vi "Firmware Wizard Config.vi"(8 "Error In":errorcluster) -> (0 "Error Out":errorcluster)   [LabVIEW 2020, in "LMH-LINX.lvlib"]
doc: "Allow user to configure settings stored in firmware wizard ini."
uses:
  LMH-LINX.lvlib
  <vilib>/Utility/config.llb/Read Key (Path).vi
  <vilib>/Utility/config.llb/Write Key (Path).vi
  <vilib>/Utility/config.llb/NI_LVConfig.lvlib
  Toolbox/LMH-Toolbox.lvlib
panel:
  in  "Generate Firmware Libs":bool
  in  "Arduino Path":path
  in  "Cancel Button":bool
  in  "Save Button":bool
  in  "Firmware Base Path":path
  # "Default Location: <LabVIEW>\\vi.lib\\MakerHub\\LINX\\Firmware\\"
  # "Default Location: <Program Files (x86)>\\Arduino"
  # "If you have the Arduino IDE, fill in the Arduino Path and use the Generate button to Generate the  firmware in the Arduino\\libraries folder\nNOTE: This will erase existing firmware in this folder"
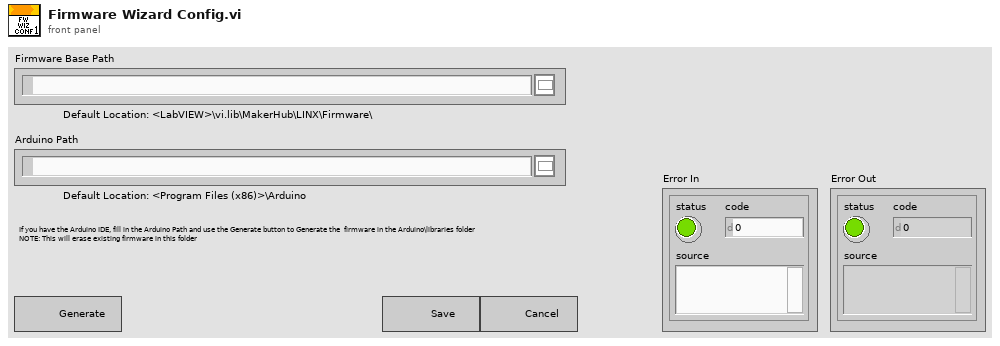
[diagram p1: front panel]
types:
  T1 = typedef "NI_LVConfig.lvlib/Config Data RefNum.ctl" = refnum<k1>
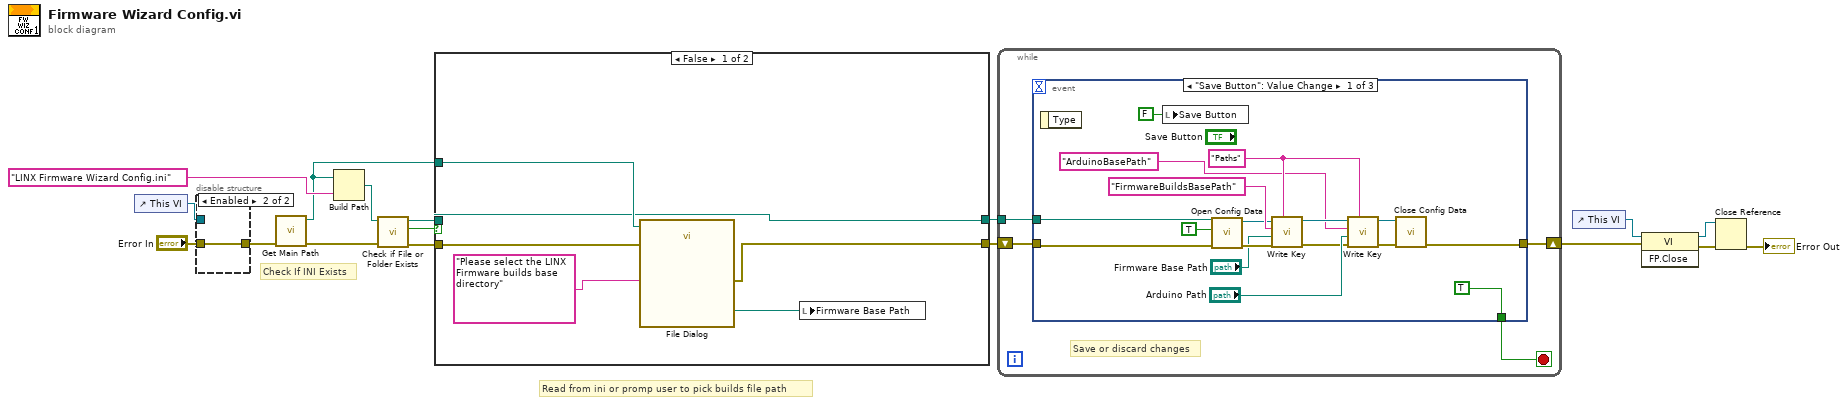
[diagram p0: block diagram]
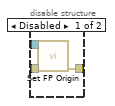
[diagram p2: hidden frame]
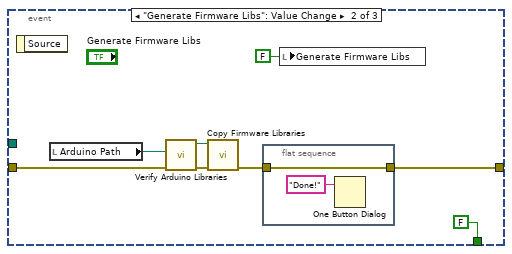
[diagram p3: hidden frame]
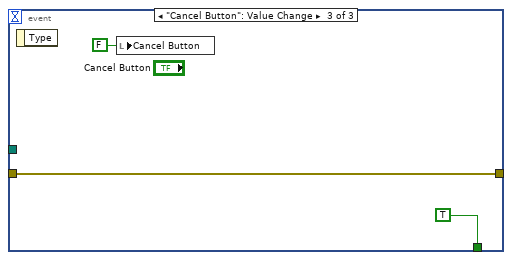
[diagram p4: hidden frame]
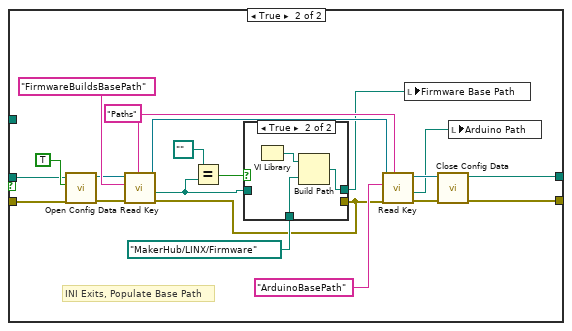
[diagram p5: hidden frame]
diagram:
  # "Read from ini or promp user to pick builds file path"
  # "Check If INI Exists"
  n1 = control-ref of="This VI"() -> (w8:refnum<vi>)
  n2 = disable-structure shown="Enabled" {
    disable-tunnel: w8 -> [w20 _]
    disable-tunnel: "Error In" -> [w19 w21]
    disable-tunnel: [w18 w21] -> w1
    frame Disabled {
      n3 = call <vilib>:"Set FP Origin.vi"("Error In"=w19, "VI Ref"=w20) -> ("Error Out"=w18:errorcluster)  [unwired: 9 in]
    }
    frame Enabled {
    }
  }
  n4 = call "Get Main Path.vi"("Error In"=w1) -> ("Error Out"=w16:errorcluster, "Main Dir"=w11:path)  [unwired: 8 in, 1 out]
  n5 = Build Path(base path=w11, name or relative path="LINX Firmware Wizard Config.ini") -> (appended path=w15:path)
  n6 = call <vilib>:"Check if File or Folder Exists.vi"("error in (no error)"=w16, "path"=w15) -> ("error out"=w12:errorcluster, "file or folder exists?"=w13:bool, "dup path"=w14:path)  [unwired: 7 in]
  n7 = case shown="False" w13 {
    tunnel: [w26 w43] -> w10
    tunnel: w14 -> [w24 w42]
    tunnel: w12 -> [w27 w41]
    tunnel: w11 -> [w25 _]
    tunnel: [w24 w40] -> w9
    frame False {
      n8 = call "File Dialog"("start path"=w25, "prompt"="Please select the LINX Firmware builds base directory", "error in"=w27) -> ("selected path"=w23:path, "error out"=w26:errorcluster)  [unwired: 9 in, 2 out]
      n9 = local write "Firmware Base Path"(w23) -> ()
    }
    frame True {
      w38 = "Paths" ("section")
      # "INI Exits, Populate Base Path"
      n10 = call <vilib>:"Open Config Data.vi"("error in (no error)"=w41, "create file if necessary (T)"=TRUE, "configuration file path"=w42) -> ("error out"=w44:errorcluster, "refnum"=w45:T1)  [unwired: 6 in, 1 out]
      n11 = call-poly <vilib>:"Read Key.vi"("section"=w38, "error in (no error)"=w44, "key"="FirmwareBuildsBasePath", "refnum"=w45) -> ("error out"=w31:errorcluster, "value"=w30:path, "refnum out"=w39:T1)  [unwired: 4 in, 1 out]
      n12 = Equal?(x=path "" ("value"), y=w30) -> (x = y?=w28:bool)
      n13 = case shown="True" w28 {
        tunnel: w31 -> [_ _]
        tunnel: path "MakerHub/LINX/Firmware" -> [_ w50]
        tunnel: w30 -> [w48 _]
        tunnel: [w48 w49] -> w32
        frame False {
        }
        frame True {
          n14 = VI Library() -> (path=w51:path)
          n15 = Build Path(base path=w51, name or relative path=w50) -> (appended path=w49:path)
        }
      }
      n16 = call-poly <vilib>:"Read Key.vi"("section"=w38, "error in (no error)"=w31, "key"="ArduinoBasePath", "refnum"=w39) -> ("error out"=w35:errorcluster, "value"=w34:path, "refnum out"=w36:T1)  [unwired: 4 in, 1 out]
      n17 = local write "Firmware Base Path"(w32) -> ()
      n18 = call <vilib>:"Close Config Data.vi"("error in (no error)"=w35, "refnum"=w36) -> ("error out"=w43:errorcluster, "file path"=w40:path)  [unwired: 8 in]
      n19 = local write "Arduino Path"(w34) -> ()
    }
  }
  n20 = while {
    tunnel: w9 -> [w54]
    shift-right: [w53] -> w3
    shift-left: w10 -> [w55]
    stop <- w52 stop-if-true
    # "Save or discard changes"
    n21 = event shown="[0] \"Save Button\": Value Change" {
      selector: _ -> [_ _ _]
      dyn-events: _ -> [_ _ _]
      timeout: _ -> [_ _ _]
      tunnel: w55 -> [w70 w80 w84]
      tunnel: [w65 w74 w84] -> w53
      tunnel: w54 -> [w67 _ _]
      tunnel: [TRUE FALSE TRUE] -> w52
      event "Save Button": Value Change {
        w62 = "Paths" ("section")
        n22 = event-data() -> ()  [unwired: 1 in, 1 out]
        n23 = local write "Save Button"(FALSE ("Save Button")) -> ()
        n24 = call <vilib>:"Open Config Data.vi"("error in (no error)"=w70, "create file if necessary (T)"=TRUE, "configuration file path"=w67) -> ("error out"=w69:errorcluster, "refnum"=w66:T1)  [unwired: 6 in, 1 out]
        n25 = call-poly <vilib>:"Write Key.vi"("section"=w62, "error in (no error)"=w69, "value"="Firmware Base Path", "key"="FirmwareBuildsBasePath", "refnum"=w66) -> ("error out"=w59:errorcluster, "refnum out"=w63:T1)  [unwired: 4 in, 1 out]
        n26 = call-poly <vilib>:"Write Key.vi"("section"=w62, "error in (no error)"=w59, "value"="Arduino Path", "key"="ArduinoBasePath", "refnum"=w63) -> ("error out"=w58:errorcluster, "refnum out"=w57:T1)  [unwired: 4 in, 1 out]
        n27 = call <vilib>:"Close Config Data.vi"("error in (no error)"=w58, "refnum"=w57) -> ("error out"=w65:errorcluster)  [unwired: 8 in, 1 out]
      }
      event "Generate Firmware Libs": Value Change {
        n28 = event-data() -> ()  [unwired: 1 in, 1 out]
        n29 = local read "Arduino Path"() -> (w79:path)
        n30 = call "Verify Arduino Libraries.vi"("Error In"=w80, "Arduino Base Path"=w79) -> ("Error Out"=w77:errorcluster, "Path to Arduino\\libraries"=w78:path)  [unwired: 7 in, 1 out]
        n31 = call "Copy Firmware Libraries.vi"("Error In"=w77, "Library Destination Dir"=w78) -> ("Error Out"=w73:errorcluster)  [unwired: 9 in]
        n32 = flat-sequence {
          tunnel: [w82] -> w74
          tunnel: w73 -> [w82]
          frame #0 {
            n33 = One Button Dialog(message="Done!") -> ()  [unwired: 1 in, 1 out]
          }
        }
        n34 = local write "Generate Firmware Libs"(FALSE ("Generate Firmware Libs")) -> ()
      }
      event "Cancel Button": Value Change {
        n35 = event-data() -> ()  [unwired: 1 in, 1 out]
        n36 = local write "Cancel Button"(FALSE ("Cancel Button")) -> ()
      }
    }
  }
  n37 = control-ref of="This VI"() -> (w4:refnum<vi>)
  n38 = invoke class="VI" method="FP.Close"(reference=w4, error in=w3) -> (reference out=w6:refnum<vi>, error out=w5:errorcluster)  [unwired: 1 in, 1 out]
  n39 = Close Reference(reference=w6, error in (no error)=w5) -> (error out=→"Error Out":errorcluster)
